vi "fpga.vi"() -> ()   [LabVIEW 2024]
uses:
  <vilib>/LabVIEW Targets/FPGA/cRIO/shared/nicrio_ModuleControls/nicrio_cRIO-9219_ConversionTime.ctl
  <vilib>/rvi/eio/common/nirviEmuTemplatePropertySet_noerrors.vi
  <vilib>/rvi/Emulation/niFpgaGetClockAttributes.vi
  <vilib>/rvi/Emulation/niFpgaSctlEmulationGetInTimedLoop.vi
  <vilib>/rvi/Emulation/niFpgaEmulationReportErrorSimple.vi
  <vilib>/rvi/eio/common/nirviEmuTemplateMethod_errors.vi
  <vilib>/rvi/Emulation/niFpgaCriticalErrorInLSC.vi
  <vilib>/eio/EIOPropertyNode/EIOPropertyNode.xnode
  <vilib>/eio/EIONode/EIONode.xnode
  <vilib>/rvi/eio/common/nirviEmuTemplatePropertyGet_errors.vi
  <vilib>/rvi/eio/common/nirviEmuTemplatePropertyGet_noerrors.vi
  <vilib>/rvi/eio/common/nirviEmuTemplatePropertySet_errors.vi
panel:
  in  "daq-period-us":u32=6000
  in  "NI-mode":T1=enum."Best 60 Hz Rejection"
  out "ch3":fxp<+,32,14>[](array[numeric])
  out "fpga-heartbeat":bool
  out "ch2":fxp<+/-,32,-1>[](array[numeric])
  out "ch1":fxp<+/-,32,-1>[](array[numeric])
  out "ch0":fxp<+/-,32,-1>[](array[numeric])
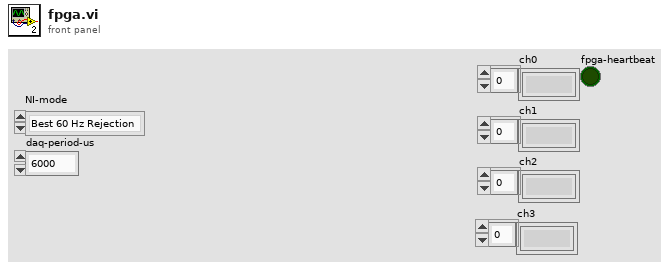
[diagram p1: front panel]
types:
  T1 = typedef "nicrio_cRIO-9219_ConversionTime.ctl" = enum8{"High Speed", "Best 60 Hz Rejection", "Best 50 Hz Rejection", "High Resolution"}
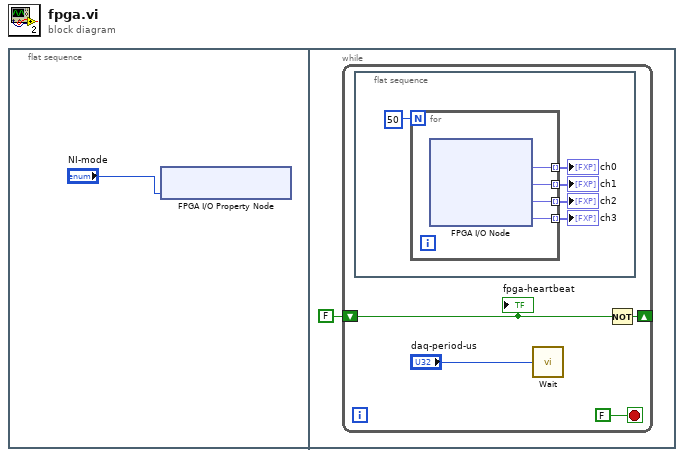
[diagram p0: block diagram]
diagram:
  n1 = flat-sequence {
    frame #0 {
      n2 = xnode "FPGA I/O Property Node"("Conversion Time"="NI-mode") -> ()  [unwired: 1 in, 1 out]
    }
    frame #1 {
      n3 = while {
        shift-right: [w3] -> _
        shift-left: FALSE -> [w4]
        stop <- FALSE stop-if-true
        n4 = flat-sequence {
          frame #0 {
            n5 = for {
              N: 50 ("nSamples") -> [_]
              tunnel: [w15] -> w10 mode=indexing
              tunnel: [w14] -> w8 mode=indexing
              tunnel: [w13] -> w9 mode=indexing
              tunnel: [w12] -> w7 mode=indexing
              n6 = xnode "FPGA I/O Node"() -> ("Mod1/CH0"=w15:fxp<+/-,32,-1>, "Mod1/CH1"=w14:fxp<+/-,32,-1>, "Mod1/CH2"=w13:fxp<+/-,32,-1>, "Mod1/CH3"=w12:fxp<+,32,14>)  [unwired: 4 in, 4 out]
            }
            "ch0" <- w10
            "ch1" <- w8
            "ch2" <- w9
            "ch3" <- w7
          }
        }
        n7 = call "Wait"("Count(mSec)"="daq-period-us") -> ()  [unwired: 1 out]
        n8 = Not(x=w4) -> (.not. x?=w3:bool)
        "fpga-heartbeat" <- w4
      }
    }
  }
